vi "Build.vi"(8 "error in (no error)":errorcluster, 11 "Build in":refnum<class "AB_EXE.lvclass">) -> (0 "error out":errorcluster, 1 "GeneratedFiles":path[](array[path]), 2 "GeneratedDirectories":path[](array[path]), 3 "Build out":refnum<class "AB_EXE.lvclass">, 4 "GeneratedFileGUIDs":string[](array[string]), 5 "OutputDirectory":path, 7 "Dependencies":T1[](array[typedef]))   [LabVIEW 2020, in "AB_EXE.lvclass"]
uses:
  <vilib>/AppBuilder/AB_Classes/EXE/AB_EXE.lvclass
  <vilib>/AppBuilder/AB_Classes/EXE/AB_EXE.lvclass/AB_EXE.ctl
  <vilib>/AppBuilder/RW_Project/AB_RW_Project_PropBag_Action.ctl
  <vilib>/AppBuilder/AB_Classes/Destination/AB_Destination.lvclass
  <vilib>/AppBuilder/AB_Classes/Application/AB_Application.lvclass
  <vilib>/AppBuilder/AB_Classes/Build/AB_Build.lvclass
  <resource>/Framework/Providers/Common/provcom_StringGlobals.vi
  <vilib>/AppBuilder/AB_Classes/TargetFile/AB_Targetfile.lvclass
  E:/2020/dist/vi.lib/AppBuilder/AB_Classes/Build/AB_Build.lvclass
  E:/2020/dist/vi.lib/AppBuilder/AB_Classes/TargetFile/AB_Targetfile.lvclass
  E:/2020/dist/vi.lib/AppBuilder/AB_Classes/Application/AB_Application.lvclass
  <vilib>/Utility/lvfile.llb/LVFileType.ctl
  <vilib>/Utility/lvfile.llb/NI_FileType.lvlib
  <vilib>/AppBuilder/AB_Dependency.ctl
panel:
  out "error out 2":errorcluster
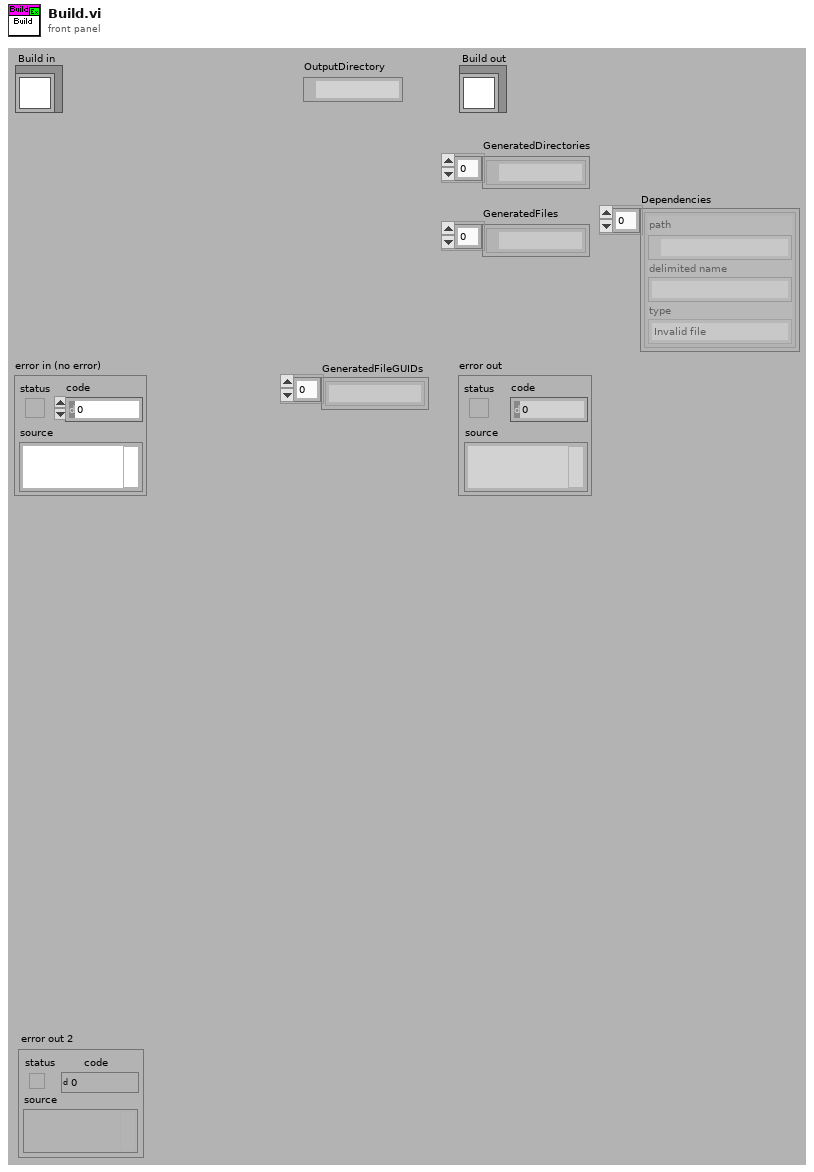
[diagram p1: front panel]
types:
  T1 = typedef "AB_Dependency.ctl" = cluster{"path":path, "delimited name":string, "type":T2}
  T2 = typedef "NI_FileType.lvlib/LVFileType.ctl" = enum32{"Invalid file", "Unknown type", "Instrument", "Control", "Polymorphic VI", "Project", "Library", "LVClass", "XControl", "XNode", "Shared library", ".NET assembly", "ActiveX interface", "CIN", "Run-time menu", "Palette menu", "Help file", "LLB", "XNode Edit Dependency", "Class Private Data Control", "Statechart", "MathScript .m file", "Ladder Diagram", "LVLibp", "XNode Build Dependency"}
  T3 = typedef "AB_RW_Project_PropBag_Action.ctl" = enum16{"read", "write", "clear", "readPrevious", "writePrevious", "clearPrevious"}
  T4 = typedef "AB_Build.ctl" = cluster{"buildSpecName":string, "buildSpecDescription":string, "destinations":refnum<class "AB_Destination.lvclass">[], "exclusionOption":T5, "defaultLanguage":string, "supportedLanguages":string[], "excludedDirectories":path[], "buildContext":refnum<vi>, "buildObject":T6, "preview":bool, "programatic":bool, "progressBarEvents":T7, "userLog_Path":path, "preActionID":string, "preAction_Path":path, "postActionID":string, "postAction_Path":path, "eng_checkForBrokenVIs?":bool, "eng_verboseLinkerErrors?":bool, "localDest_Path":path, "targetDest_Path":path, "removeVIObject":u16, "cache":refnum<class "PreviewCache.lvclass">, "use cache":bool, "previewCache_ID":string, "buildCache_ID":string, "eng_TempLocalDest_Path":path, "eng_collectDependencies?":bool, "versionInfo":cluster{"buildVersion":cluster{"major":u16, "minor":u16, "patch":u16, "build":u16}, "autoIncrement":bool}, "eng_enableVIChecksums":bool}
  T5 = typedef "AB_Exclusion_Option.ctl" = cluster{"typedefs":bool, "polymorphicVIs":bool, "unusedLibraryItems":bool, "modifyLibraryFile":bool, "edit-timeDependencies":bool, "inlineVIs":bool, "dependent PPLs":bool, "dependent DLLs":bool}
  T6 = typedef "ItemRef.ctl" = u64
  T7 = typedef "provcom_ProgressBar_Events.ctl" = cluster{"newJob":refnum<user-event>, "newItem":refnum<user-event>, "errorMsg":T8, "cancel":refnum<user-event>}
  T8 = typedef "mxLvBuildError.ctl" = refnum<user-event>
  T9 = typedef "AB_CopyFiles_Data.ctl" = cluster{"processedItems":T10[]}
  T10 = typedef "AB_Source_Processed_Info.ctl" = cluster{"destPath":path, "buildDelimitedName":string, "sourceIndex":i32, "topLevel":bool}
  T11 = typedef "AB_Targetfile.ctl" = cluster{"targetfileName":string, "targetfileGUID":string, "enableDebugging":bool, "versionInfo":cluster{"productName":string, "legalCopyright":string, "companyName":string, "internalName":string, "fileDescription":string}, "eng_consolidatedTypeInfo":string, "fastFileFormat":bool, "eng_LEIFBuildData":u32, "versionIndependent":bool}
  T12 = typedef "AB_Application.ctl" = cluster{"INI_path":path, "INI_itemID":string, "INI_GUID":string, "aliasPath":path, "aliasItemID":string, "aliasGUID":string, "waitDebugging":bool, "copyErrors":bool, "useFFRTE":bool, "includeHWConfig":bool, "showHWConfig":bool, "winsec.certificate":string, "winsec.timestamp":string, "winsec.description":string, "winsec.manifestItemID":string, "winsec.manifestPath":path, "web service itemIDs":string[], "Embedded Server Configuration":T13, "Server Type":enum32{"NI Web Server", "Application Web Server"}}
  T13 = typedef "AB_Embedded_Server_Configuration.ctl" = cluster{"HTTP enabled?":bool, "HTTP port":i32, "HTTPS enabled?":bool, "HTTPS port":i32, "SSL certificate file":path}
  T14 = typedef "AB_Destination.ctl" = cluster{"destName":string, "path":path, "libraryName":string, "preserveHierarchy":bool, "eng_inBuild":bool, "eng_libraryReference":refnum<vi>, "eng_restictAddToNewLibrary":bool}
  T15 = enum32{"invalid OS target", "Mac OS", "Windows 3.1", "Windows 95/NT", "Solaris 1", "Solaris 2", "HP-UX", "PowerMAX", "Linux", "Irix", "Rhapsody", "BeOS", "AIX", "OSF1", "VxWorks", "PharLap", "Carbon", "RTX", "Windows x64", "Linux x64", "Mac OS X x64"}
  T16 = typedef "AB_Engine_RTDEP_LibDeploymentInfo.ctl" = cluster{"auto undeploy?":bool, "Array":T17[], "hide deployment dialog":bool}
  T17 = typedef "AB_Engine_RTDEP_Dep_Lib_Info.ctl" = cluster{"Library Path":path, "Target Name":string}
  T18 = typedef "AB_Version_Info.ctl" = cluster{"PrivateBuild":string, "SpecialBuild":string, "LegalCopyright":string, "LegalTrademarks":string, "Comments":string, "FileDescription":string, "InternalName":string, "file version":cluster{"major":u16, "minor":u16, "patch":u16, "build":u16}, "ProductName":string, "FileType":u16, "CompanyName":string, "OriginalFilename":string}
  T19 = typedef "AB_RW_Project_EXE_ActiveX_Data.ctl" = cluster{"Major Version":u16, "Minor Version":u16, "ProgID Prefix":string, "Obj CLSIDs":string[], "Enum CLSIDs":string[]}
  T20 = cluster{"appended path":path, "appended path":path, "actXServerName":string, "App Memory Size":u32, "LVRT Target Dialog":i32, "pathAppShell":path, "AppFlags":u32, "activeX info out":T19, "empty":bool, "defaultLanguage":string, "supportedLanguages":string[], "Lib Deployment Info":T16, "eng_consolidatedTypeInfo":string, "eng_LEIFBuildData":u32}
  T21 = cluster{"Major Version":u16, "Minor Version":u16, "ProgID Prefix":string, "Obj CLSIDs":string[], "Enum CLSIDs":string[]}
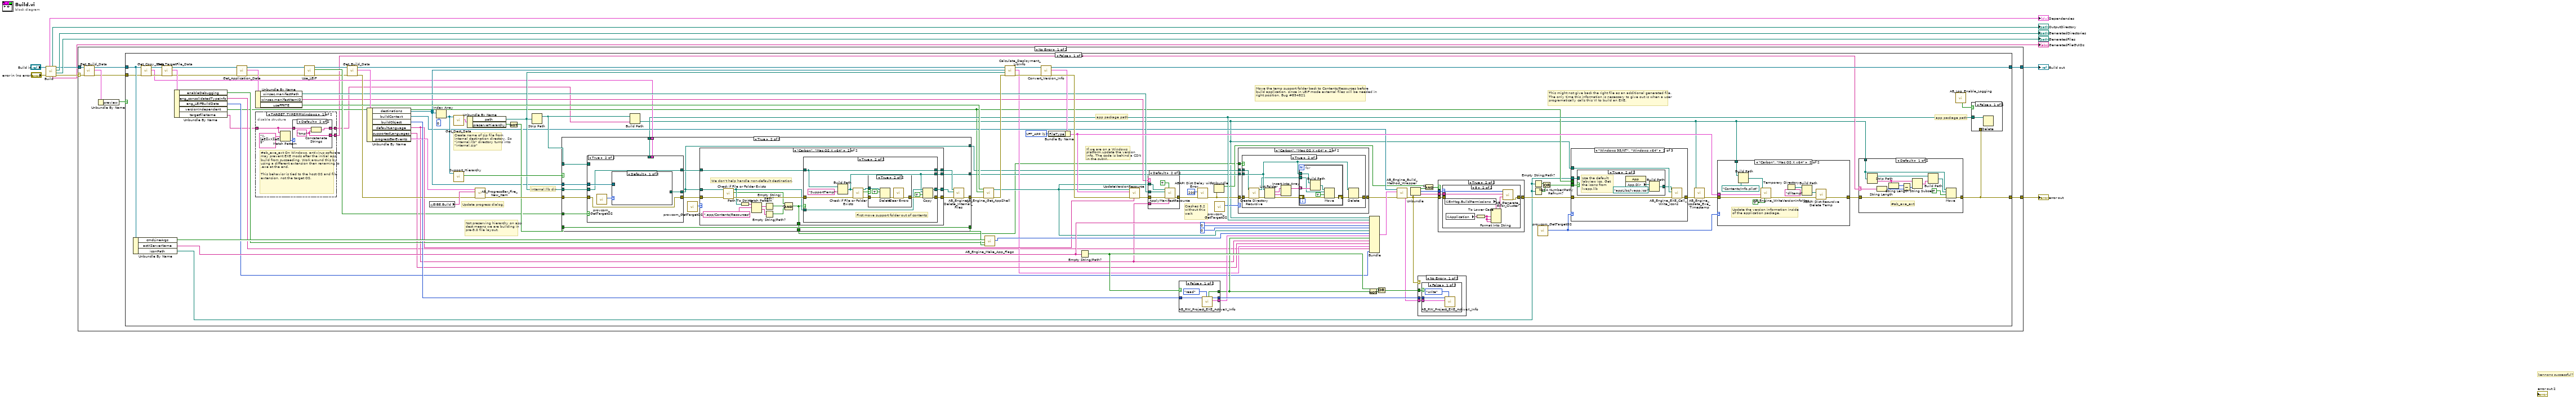
[diagram p0: block diagram]
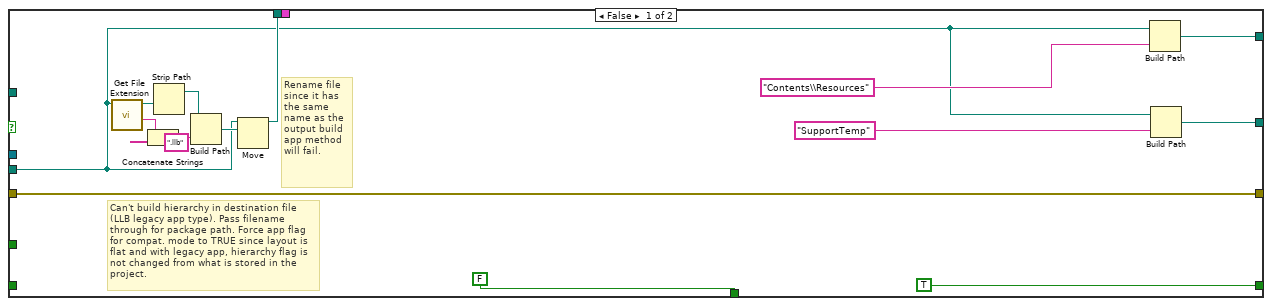
[diagram p8: hidden frame]
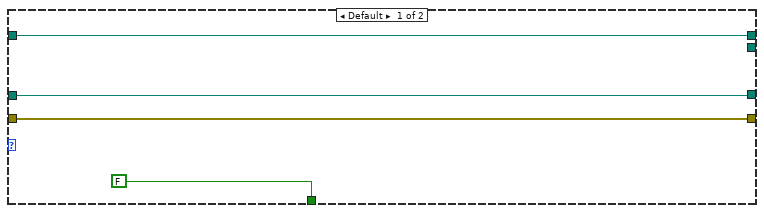
[diagram p9: hidden frame]
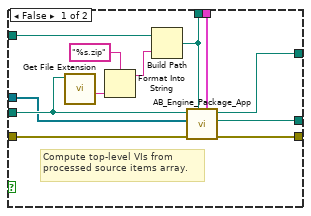
[diagram p12: hidden frame]
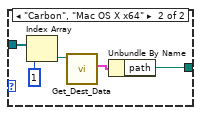
[diagram p13: hidden frame]
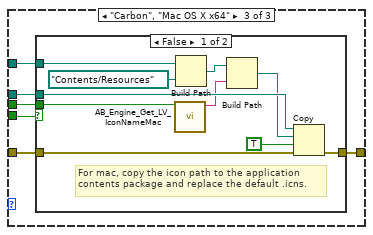
[diagram p18: hidden frame]
diagram:
  # "kennonc successful?"
  n1 = call-parent "Build.vi"("error in (no error)"="error in (no error)", "Build in"="Build in") -> ("error out"=w4:errorcluster, "GeneratedFiles"=→"GeneratedFiles":path[], "GeneratedDirectories"=→"GeneratedDirectories":path[], "Build out"=w5:refnum<class "AB_EXE.lvclass">, "GeneratedFileGUIDs"=→"GeneratedFileGUIDs":string[], "OutputDirectory"=→"OutputDirectory":path, "Dependencies"=→"Dependencies":T1[])  [unwired: 3 out]
  n2 = case shown="No Error" w4 {
    selector: w4 -> [w13 w338]
    tunnel: [w19 w336] -> w7
    tunnel: [w18 w337] -> w6
    tunnel: w5 -> [w17 w339]
    frame No Error {
      n3 = call <vilib>:"Get_Build_Data.vi"("error in (no error)"=w13, "Class in"=w17) -> ("error out"=w12:errorcluster, "data"=w16:T4, "Class out"=w14:refnum<class "AB_EXE.lvclass">)  [unwired: 7 out]
      n4 = Unbundle By Name(w16) -> ("preview"=w15:bool)
      n5 = case shown="False" w15 {
        tunnel: [w59 w335] -> w19
        tunnel: [w22 w334] -> w18
        tunnel: w14 -> [w64 w335]
        tunnel: w12 -> [w62 w334]
        frame False {
          w97 = u16 1 items=["VFT_UNKNOWN", "VFT_APP", "VFT_DLL", "VFT_DRV", "VFT_FONT", "VFT_VXD", "-", "VFT_STATIC_LIB"] ("FileType")
          # "Move the temp support folder back to Contents/Resources before build application, since in LEIF mode external files will be needed in right position. Bug #894821"
          # "Not preserving hierarchy on app dest means we are building in pre-9.0 file layout."
          # "Create name of zip file from internal destination directory. So \"internal.llb\" directory turns into \"internal.zip\""
          # "internal.llb dir"
          # "app package path"
          # "app package path"
          # "Update progress dialog."
          # "If we are on a Windows platform,update the version info. The code is behind a CDN in the subVI."
          # "Crashes 8.2 without this wait"
          # "This might not give back the right file as an additional generated file.\nThe only time this information is necessary to give out is when a user\nprogramatically calls this VI to build an EXE."
          n6 = Unbundle By Name(w64) -> ("cmdLineArgs"=w110:bool, "actXServerName"=w54:string, "iconPath"=w34:path)
          n7 = call <vilib>:"Get_Copy_Data.vi"("error in (no error)"=w62, "AB_Build in"=w64) -> ("error out"=w61:errorcluster, "copyData"=w60:T9, "AB_Build out"=w63:refnum<class "AB_EXE.lvclass">)  [unwired: 7 in]
          n8 = call <vilib>:"Get_TargetFile_Data.vi"("error in (no error)"=w61, "AB_Targetfile in"=w63) -> ("error out"=w39:errorcluster, "data"=w67:T11, "AB_Targetfile out"=w66:refnum<class "AB_EXE.lvclass">)  [unwired: 7 in]
          n9 = Unbundle By Name(w67) -> ("enableDebugging"=w65:bool, "eng_consolidatedTypeInfo"=w44:string, "eng_LEIFBuildData"=w38:u32, "versionIndependent"=w35:bool, "targetfileName"=w25:string)
          n10 = call <vilib>:"Get_Application_Data.vi"("error in (no error)"=w39, "AB_Application in"=w66) -> ("error out"=w40:errorcluster, "data"=w102:T12, "AB_Application out"=w42:refnum<class "AB_EXE.lvclass">)  [unwired: 7 out]
          n11 = Unbundle By Name(w102) -> ("winsec.manifestPath"=w73:path, "winsec.manifestItemID"=w72:string, "useFFRTE"=w87:bool)
          n12 = disable-structure shown="TARGET_TYPE==Windows" {
            disable-tunnel: [w133 w138] -> w20
            disable-tunnel: [w132 _] -> w24
            disable-tunnel: w25 -> [w131 w138]
            frame condition #0 (active) {
              # "#ab_exe_ext On Windows, antivirus software may prevent EXE mods after the initial app build from succeeding. Work around this by using a different extension then renaming to .exe at the end.\n\nThis behavior is tied to the host OS and file extension, not the target OS."
              n13 = Match Pattern(string=w131, regular expression="\\.[eE][xX][eE]$") -> (offset past match=w129:i32)  [unwired: 1 in, 3 out]
              n14 = case shown="Default" w129 {
                tunnel: [w134 w137] -> w133
                tunnel: [_ w136] -> w132
                tunnel: w131 -> [w134 w135]
                frame -1 {
                }
                frame Default {
                  w136 = "tmp" ("string")
                  n15 = Concatenate Strings(w135, w136) -> (w137:string)
                }
              }
            }
            frame condition #1 {
            }
          }
          n16 = call <vilib>:"Use_LEIF.vi"("error in (no error)"=w40, "AB_Targetfile in"=w42) -> ("error out"=w36:errorcluster, "use LEIF?"=w41:bool, "AB_Targetfile out"=w37:refnum<class "AB_EXE.lvclass">)  [unwired: 7 in]
          n17 = call <vilib>:"Get_Build_Data.vi"("error in (no error)"=w36, "Class in"=w37) -> ("error out"=w86:errorcluster, "data"=w101:T4, "Class out"=w79:refnum<class "AB_EXE.lvclass">)  [unwired: 7 out]
          n18 = Unbundle By Name(w101) -> ("destinations"=w68:refnum<class "AB_Destination.lvclass">[], "buildContext"=w58:refnum<vi>, "buildObject"=w100:T6, "defaultLanguage"=w47:string, "supportedLanguages"=w46:string[], "progressBarEvents"=w94:T7)
          n19 = global read "provcom_StringGlobals.vi" "EIBE.Build"() -> (w95:string)
          n20 = Index Array(array=w68, index=0) -> (element=w82:refnum<class "AB_Destination.lvclass">)
          n21 = call <vilib>:"Get_Dest_Data.vi"("Class in"=w82) -> ("destName"=w104:T14)  [unwired: 1 in, 9 out]
          n22 = call-dynamic "Support_Hierarchy.vi"("AB_Destination in"=w82) -> ("support hierarchy"=w81:bool)  [unwired: 8 in, 2 out]
          n23 = Unbundle By Name(w104) -> ("path"=w76:path, "preserveHierarchy"=w71:bool)
          n24 = call <vilib>:"AB_ProgressBar_Fire_New_Item.vi"("error in (no error)"=w86, "Label"=w95, "progressBarEvents in"=w94) -> ("error out"=w85:errorcluster)  [unwired: 8 out]
          n25 = Not(x=w71) -> (.not. x?=w70:bool)
          n26 = Strip Path(path=w76) -> (stripped path=w83:path)  [unwired: 1 out]
          n27 = case shown="True" w81 {
            tunnel: w85 -> [w185 w203]
            tunnel: [w185 w196] -> w84
            tunnel: w76 -> [w173 w200]
            tunnel: w83 -> [_ w202]
            tunnel: [w178 w201] -> w55
            tunnel: w70 -> [_ w199]
            tunnel: [TRUE w199] -> w69
            tunnel: w68 -> [_ w198]
            tunnel: w60 -> [_ w197]
            tunnel: w41 -> [_ w195]
            tunnel: [w175 w187] -> w32
            tunnel: [w174 w190] -> w33
            tunnel: [FALSE ("file or folder exists?") w186] -> w27
            frame False {
              # "Rename file since it has the same name as the output build app method will fail."
              # "Can't build hierarchy in destination file (LLB legacy app type). Pass filename through for package path. Force app flag for compat. mode to TRUE since layout is flat and with legacy app, hierarchy flag is not changed from what is stored in the project."
              n28 = call <vilib>:"Get File Extension.vi"("file"=w173) -> ("filename without extension"=w179:string, "dup file"=w181:path)  [unwired: 1 in, 8 out]
              n29 = Concatenate Strings(w179, ".llb" ("string")) -> (w182:string)
              n30 = Strip Path(path=w181) -> (stripped path=w177:path)  [unwired: 1 out]
              n31 = Build Path(base path=w177, name or relative path=w182) -> (appended path=w183:path)
              n32 = Move(source path=w173, 10:w183) -> (3:w178:path)  [unwired: 1 in, 4 out]
              n33 = Build Path(base path=w173, name or relative path="Contents\\Resources") -> (appended path=w175:path)
              n34 = Build Path(base path=w173, name or relative path="SupportTemp") -> (appended path=w174:path)
            }
            frame True {
              n35 = case shown="True" w195 {
                tunnel: w203 -> [w257 w262]
                tunnel: w202 -> [w253 _]
                tunnel: [w252 _] -> w201
                tunnel: [w246 w262] -> w188
                tunnel: w200 -> [w251 w258]
                tunnel: w198 -> [w250 w260]
                tunnel: w197 -> [w249 _]
                tunnel: [w248 w258] -> w194
                tunnel: [w247 w259] -> w187
                frame False {
                  # "Compute top-level VIs from processed source items array."
                  n36 = call <vilib>:"Get File Extension.vi"("file"=w251) -> ("filename without extension"=w256:string)  [unwired: 1 in, 9 out]
                  n37 = Format Into String(format string="%s.zip", w256) -> (resulting string=w255:string)  [unwired: 2 in, 1 out]
                  n38 = Build Path(base path=w253, name or relative path=w255) -> (appended path=w252:path)
                  n39 = call <vilib>:"AB_Engine_Package_App.vi"("processed_sourceItems"=w249, "application package path"=w252, "error in (no error)"=w257, "destinations"=w250, "internal directory"=w251) -> ("error out"=w246:errorcluster, "support dir"=w247:path, "dup internal directory"=w248:path)  [unwired: 1 in, 3 out]
                }
                frame True {
                  n40 = call <resource>:"provcom_GetTargetOS.vi"() -> ("App.TargetOS"=w261:T15)  [unwired: 11 out]
                  n41 = case shown="Default" w261 {
                    tunnel: w260 -> [_ w264]
                    tunnel: [_ w263] -> w259
                    frame Default {
                    }
                    frame "Carbon", "Mac OS X x64" {
                      n42 = Index Array(array=w264, index=1) -> (element=w267:refnum<class "AB_Destination.lvclass">)
                      n43 = call <vilib>:"Get_Dest_Data.vi"("Class in"=w267) -> ("destName"=w266:T14)  [unwired: 1 in, 9 out]
                      n44 = Unbundle By Name(w266) -> ("path"=w263:path)
                    }
                  }
                }
              }
              n45 = call <resource>:"provcom_GetTargetOS.vi"() -> ("App.TargetOS"=w189:T15)  [unwired: 11 out]
              n46 = case shown="\"Carbon\", \"Mac OS X x64\"" w189 {
                tunnel: w194 -> [w207 w224]
                tunnel: [w205 w223] -> w193
                tunnel: [w204 w222] -> w192
                tunnel: [w207 w221] -> w191
                tunnel: [_ w220] -> w190
                tunnel: w188 -> [w204 w219]
                tunnel: w187 -> [w205 w218]
                tunnel: [FALSE ("file or folder exists?") w211] -> w186
                frame Default {
                }
                frame "Carbon", "Mac OS X x64" {
                  # "We don't help handle non-default destination."
                  n47 = call <vilib>:"Check if File or Folder Exists.vi"("error in (no error)"=w219, "path"=w218) -> ("error out"=w217:errorcluster, "file or folder exists?"=w212:bool, "dup path"=w215:path)  [unwired: 7 in]
                  n48 = Path To String(path=w215) -> (string=w216:string)
                  n49 = Match Pattern(string=w216, regular expression=".app/Contents/Resources") -> (match substring=w213:string, after substring=w210:string)  [unwired: 1 in, 2 out]
                  n50 = Empty String/Path?(string/path=w213) -> (empty?=w209:bool)
                  n51 = Empty String/Path?(string/path=w210) -> (empty?=w208:bool)
                  n52 = Compound Arithmetic op=AND(w212, invert w209, w208) -> (w211:bool)
                  n53 = case shown="True" w211 {
                    tunnel: w217 -> [w225 w239]
                    tunnel: w224 -> [w227 w229]
                    tunnel: w215 -> [w226 w232]
                    tunnel: [w226 w231] -> w223
                    tunnel: [w225 w230] -> w222
                    tunnel: [w227 w229] -> w221
                    tunnel: [_ w228] -> w220
                    frame False {
                    }
                    frame True {
                      # "First move support folder out of contents"
                      n54 = Build Path(base path=w229, name or relative path="SupportTemp") -> (appended path=w228:path)
                      n55 = call <vilib>:"Check if File or Folder Exists.vi"("error in (no error)"=w239, "path"=w228) -> ("error out"=w236:errorcluster, "file or folder exists?"=w237:bool, "dup path"=w235:path)  [unwired: 7 in]
                      n56 = case shown="True" w237 {
                        tunnel: w236 -> [w240 w245]
                        tunnel: [w240 w242] -> w234
                        tunnel: w235 -> [_ w241]
                        frame False {
                        }
                        frame True {
                          n57 = Delete(path (use dialog)=w241, entire hierarchy (F)=TRUE, error in=w245) -> (error out=w243:errorcluster)  [unwired: 2 in, 2 out]
                          n58 = call <vilib>:"Clear Errors.vi"("error in (no error)"=w243) -> ("error out"=w242:errorcluster)  [unwired: 5 in, 1 out]
                        }
                      }
                      n59 = Copy(8:w234, 9:TRUE ("overwrite (F)"), 10:w228, 11:w232) -> (0:w230:errorcluster, 3:w231:path)  [unwired: 1 in, 1 out]
                    }
                  }
                }
              }
              n60 = call <vilib>:"AB_Engine_Delete_Internal_Files.vi"("error in (no error)"=w192, "support dir"=w193, "internal directory"=w191) -> ("error out"=w196:errorcluster)  [unwired: 8 in]
            }
          }
          n61 = Build Path(base path=w83, name or relative path=w20) -> (appended path=w21:path)
          n62 = call <vilib>:"AB_Engine_Get_AppShell.vi"("error in (no error)"=w84, "useBCRTE"=w35, "useFFRTE"=w87) -> ("error out"=w80:errorcluster, "pathAppShell"=w51:path)  [unwired: 7 out]
          n63 = call <vilib>:"AB_Engine_Make_App_Flags.vi"("App Compatibility Mode"=w69, "enable debugging"=w65, "cmd line arg"=w110) -> ("AppFlags"=w50:u32)  [unwired: 8 in]
          n64 = call <vilib>:"Calculate_Deployment_LibInfo.vi"("error in (no error)"=w80, "main destination"=w76, "destinations"=w68, "AB_EXE in"=w79) -> ("error out"=w77:errorcluster, "Lib Deployment Info"=w45:T16, "AB_EXE out"=w78:refnum<class "AB_EXE.lvclass">)  [unwired: 5 out]
          n65 = call-dynamic "Convert_Version_Info.vi"("error in (no error)"=w77, "AB_Targetfile in"=w78) -> ("error out"=w98:errorcluster, "input version info"=w96:T18, "AB_Targetfile out"=w59:refnum<class "AB_EXE.lvclass">)  [unwired: 7 out]
          n66 = Bundle By Name(cluster=w96, "FileType"=w97) -> (w93:T18)
          n67 = Empty String/Path?(string/path=w54) -> (empty?=w108:bool)
          n68 = call <resource>:"UpdateVersionResource.vi"("default language"=w47, "error in (no error)"=w98, "input version info"=w93, "path"=w51) -> ("error out"=w75:errorcluster)  [unwired: 1 in, 6 out]
          n69 = case shown="Default" w72 {
            tunnel: w75 -> [w164 w170]
            tunnel: [w164 w169] -> w74
            tunnel: w51 -> [_ w168]
            tunnel: w47 -> [_ w167]
            tunnel: w73 -> [_ w166]
            frame "" {
            }
            frame Default {
              n70 = call <resource>:"ApplyManifestResource.vi"("default language"=w167, "remove English resource?"=TRUE, "error in (no error)"=w170, "manifest path"=w166, "path"=w168) -> ("error out"=w169:errorcluster)  [unwired: 6 in]
            }
          }
          n71 = case shown="False" w108 {
            tunnel: w100 -> [w319 w320]
            tunnel: [w317 _] -> w49
            tunnel: [w316 _] -> w48
            tunnel: [w315 w320] -> w106
            frame False {
              n72 = call <vilib>:"AB_RW_Project_EXE_ActiveX_Info.vi"("action"=AB_RW_Project_PropBag_Action."read", "Object In"=w319) -> ("activeX info out"=w317:T19, "Object Out"=w315:T6, "empty"=w316:bool)  [unwired: 2 in, 5 out]
            }
            frame True {
            }
          }
          n73 = call <vilib>:"ABAPI Dist Delay with Error.vi"("error in (no error)"=w74, "milliseconds to wait"=u32 200) -> ("error out"=w31:errorcluster)  [unwired: 1 in, 8 out]
          n74 = Unbundle(w31) -> ("status"=w29:bool)  [unwired: 2 out]
          n75 = call <resource>:"provcom_GetTargetOS.vi"() -> ("App.TargetOS"=w28:T15)  [unwired: 11 out]
          n76 = case shown="\"Carbon\", \"Mac OS X x64\"" w28 {
            tunnel: w27 -> [_ w144]
            tunnel: w33 -> [_ w143]
            tunnel: w32 -> [_ w142]
            tunnel: w31 -> [w139 w141]
            tunnel: [w139 w140] -> w30
            frame Default {
            }
            frame "Carbon", "Mac OS X x64" {
              n77 = case shown="True" w144 {
                tunnel: w141 -> [w145 w149]
                tunnel: [w145 w152] -> w140
                tunnel: w143 -> [_ w150]
                tunnel: w142 -> [_ w147]
                frame False {
                }
                frame True {
                  n78 = call <vilib>:"Create Directory Recursive.vi"("error in (no error)"=w149, "directory"=w147) -> ("error out"=w148:errorcluster, "directory copy"=w146:path)  [unwired: 3 in, 1 out]
                  n79 = List Folder(path=w150, error in=w148) -> (filenames=w155:string[], folder names=w156:string[], error out=w154:errorcluster)  [unwired: 2 in, 1 out]
                  n80 = Insert Into Array(array=w155, new element=w156) -> (w151:string[])  [unwired: 1 in]
                  n81 = for {
                    shift-right: [w160] -> w153
                    shift-left: w154 -> [w163]
                    tunnel: w151 -> [w162] mode=indexing
                    tunnel: w150 -> [w161]
                    tunnel: w146 -> [w157]
                    n82 = Build Path(base path=w161, name or relative path=w162) -> (appended path=w158:path)
                    n83 = Move(source path=w158, error in=w163, 9:TRUE ("overwrite (F)"), 10:w157) -> (error out=w160:errorcluster)  [unwired: 1 in, 2 out]
                  }
                  n84 = Delete(path (use dialog)=w150, error in=w153) -> (error out=w152:errorcluster)  [unwired: 3 in, 2 out]
                }
              }
            }
          }
          n85 = Not(x=w48) -> (.not. x?=w105:bool)
          n86 = Bundle("appended path"=w21, "appended path"=w55, "actXServerName"=w54, "App Memory Size"=u32 0, "LVRT Target Dialog"=0, "pathAppShell"=w51, "AppFlags"=w50, "activeX info out"=w49, "empty"=w48, "defaultLanguage"=w47, "supportedLanguages"=w46, "Lib Deployment Info"=w45, "eng_consolidatedTypeInfo"=w44, "eng_LEIFBuildData"=w38) -> (w43:T20)  [unwired: 1 in]
          n87 = Or(x=w108, y=w105) -> (x .or. y?=w107:bool)
          n88 = call <vilib>:"AB_Engine_Build_Method_Wrapper.vi"("error in"=w30, "build cluster"=w43, "buildContext"=w58) -> ("error out"=w56:errorcluster, "axInfo"=w57:T21)  [unwired: 7 in]
          n89 = Unbundle(w56) -> ("status"=w92:bool, "code"=w90:i32, "source"=w88:string)
          n90 = case shown="No Error" w56 {
            tunnel: w107 -> [w311 _]
            tunnel: w106 -> [w310 _]
            tunnel: w57 -> [w309 _]
            frame No Error {
              n91 = case shown="False" w311 {
                tunnel: w310 -> [w314 _]
                tunnel: w309 -> [w312 _]
                frame False {
                  n92 = call <vilib>:"AB_RW_Project_EXE_ActiveX_Info.vi"("action"=AB_RW_Project_PropBag_Action."write", "activeX info in"=w312, "Object In"=w314) -> ()  [unwired: 1 in, 8 out]
                }
                frame True {
                }
              }
            }
            frame Error {
            }
          }
          n93 = Compound Arithmetic op=AND(invert w29, w92) -> (w91:bool)
          n94 = case shown="True" w91 {
            tunnel: w56 -> [w268 w271]
            tunnel: w90 -> [_ w272]
            tunnel: [w268 w270] -> w89
            tunnel: w88 -> [_ w269]
            frame False {
            }
            frame True {
              n95 = case shown="8" w272 {
                selector: w272 -> [_ w280]
                tunnel: w271 -> [w273 _]
                tunnel: [w273 w278] -> w270
                tunnel: w269 -> [_ w279]
                frame Default {
                }
                frame 8 {
                  n96 = global read "provcom_StringGlobals.vi" "ErrMsg.BuildPermissions"() -> (w276:string)
                  n97 = global read "provcom_StringGlobals.vi" "Application"() -> (w275:string)
                  n98 = To Lower Case(string=w275) -> (all lower case string=w277:string)
                  n99 = Format Into String(format string=w276, w277, w277, w277) -> (resulting string=w274:string)  [unwired: 2 in, 1 out]
                  n100 = call <vilib>:"AB_Generate_Error_Cluster.vi"("Additional Message"=w274, "source"=w279, "Code"=w280) -> ("error out"=w278:errorcluster)  [unwired: 1 in, 7 out]
                }
              }
            }
          }
          n101 = Empty String/Path?(string/path=w34) -> (empty?=w115:bool)
          n102 = Not A Number/Path/Refnum?(number/path/refnum=w34) -> (NaN/Path/Refnum?=w114:bool)
          n103 = call <resource>:"provcom_GetTargetOS.vi"() -> ("App.TargetOS"=w26:T15)  [unwired: 11 out]
          n104 = Or(x=w115, y=w114) -> (x .or. y?=w99:bool)
          n105 = case shown="\"Windows 95/NT\", \"Windows x64\"" w26 {
            tunnel: w89 -> [w281 w287 w292]
            tunnel: w34 -> [_ w284 w293]
            tunnel: [w281 w286 w297] -> w112
            tunnel: w21 -> [_ w285 w294]
            tunnel: w99 -> [_ w282 w295]
            tunnel: w35 -> [_ _ w296]
            frame Default {
            }
            frame "Windows 95/NT", "Windows x64" {
              n106 = case shown="True" w282 {
                tunnel: [w288 w291] -> w283
                tunnel: w284 -> [w288 _]
                frame False {
                }
                frame True {
                  # "Use the default labview ico. Get the icons from lvapp.lib"
                  n107 = property class="App"() -> ("App.Dir"=w289:path)  [unwired: 2 in, 2 out]
                  n108 = Build Path(base path=w289, name or relative path=path "appLibs/lvapp.ico") -> (appended path=w291:path)
                }
              }
              n109 = call <vilib>:"AB_Engine_EXE_Call_Write_Icons.vi"("error in (no error)"=w287, "application path"=w285, "icon path"=w283) -> ("error out"=w286:errorcluster)  [unwired: 8 out]
            }
            frame "Carbon", "Mac OS X x64" {
              n110 = case shown="False" w295 {
                tunnel: w292 -> [w307 w308]
                tunnel: w293 -> [w306 _]
                tunnel: [w305 w308] -> w297
                tunnel: w294 -> [w304 _]
                tunnel: w296 -> [w298 _]
                frame False {
                  # "For mac, copy the icon path to the application\ncontents package and replace the default .icns."
                  n111 = call <vilib>:"AB_Engine_Get_LV_IconNameMac.vi"("use version independent app"=w298) -> ("icon file name"=w299:string)  [unwired: 1 in, 9 out]
                  n112 = Build Path(base path=w304, name or relative path=path "Contents/Resources") -> (appended path=w301:path)
                  n113 = Build Path(base path=w301, name or relative path=w299) -> (appended path=w300:path)
                  n114 = Copy(8:w307, 9:TRUE ("overwrite (F)"), 10:w300, 11:w306) -> (0:w305:errorcluster)  [unwired: 3 out]
                }
                frame True {
                }
              }
            }
          }
          n115 = call <vilib>:"AB_Engine_Update_Exe_Timestamp.vi"("error in (no error)"=w112, "pathExe"=w21) -> ("error out"=w111:errorcluster)  [unwired: 9 out]
          n116 = case shown="\"Carbon\", \"Mac OS X x64\"" w26 {
            tunnel: w111 -> [w321 w330]
            tunnel: [w321 w324] -> w23
            tunnel: w93 -> [_ w329]
            tunnel: w21 -> [_ w323]
            frame Default {
            }
            frame "Carbon", "Mac OS X x64" {
              # "Update the version information inside\nof the application package."
              n117 = Build Path(base path=w323, name or relative path=path "Contents/Info.plist") -> (appended path=w332:path)
              n118 = call <vilib>:"AB_Engine_WriteVersionInfoMac.vi"("set CFBundleIdentifier"=TRUE, "error in (no error)"=w330, "version info"=w329, "FilePath"=w332) -> ("error out"=w325:errorcluster)  [unwired: 7 out]
              n119 = Temporary Directory() -> (w326:path)
              n120 = Build Path(base path=w326, name or relative path="dlltemp") -> (appended path=w328:path)
              n121 = call <vilib>:"ABAPI Dist Recursive Delete Temp.vi"("error in (no error)"=w325, "path"=w328) -> ("error out"=w324:errorcluster)  [unwired: 1 out]
            }
          }
          n122 = case shown="Default" w24 {
            selector: w24 -> [w116 _]
            tunnel: w23 -> [w119 w128]
            tunnel: [w118 w128] -> w22
            tunnel: w21 -> [w117 _]
            frame Default {
              # "#ab_exe_ext"
              n123 = Strip Path(path=w117) -> (stripped path=w124:path, name=w121:string)
              n124 = String Length(string=w116) -> (length=w122:i32)
              n125 = String Length(string=w121) -> (length=w123:i32)
              n126 = Subtract(x=w123, y=w122) -> (x-y=w120:i32)
              n127 = String Subset(string=w121, length (rest)=w120) -> (substring=w125:string)  [unwired: 1 in]
              n128 = Build Path(base path=w124, name or relative path=w125) -> (appended path=w127:path)
              n129 = Move(source path=w117, error in=w119, 9:TRUE ("overwrite (F)"), 10:w127) -> (error out=w118:errorcluster)  [unwired: 1 in, 2 out]
            }
            frame "" {
            }
          }
          n130 = call <vilib>:"AB_Log_Enable_Logging.vi"() -> ("keep internal.llb"=w103:bool)  [unwired: 2 in, 9 out]
          n131 = case shown="False" w103 {
            tunnel: w22 -> [_ _]
            tunnel: w55 -> [w333 _]
            frame False {
              n132 = Delete(path (use dialog)=w333) -> ()  [unwired: 4 in, 3 out]
            }
            frame True {
            }
          }
        }
        frame True {
        }
      }
    }
    frame Error {
      n133 = call-dynamic "Delete_Internal_TargetFileDir_On_Error.vi"("error in (no error)"=w338, "Build in"=w339) -> ("error out"=w337:errorcluster, "Build out"=w336:refnum<class "AB_EXE.lvclass">)  [unwired: 8 in]
    }
  }
  "error out" <- w6
  "Build out" <- w7
